vi "VIP_Post-Install Custom Action.vi"(10 "Variant":variant) -> (0 "error out":errorcluster)   [LabVIEW 2020]
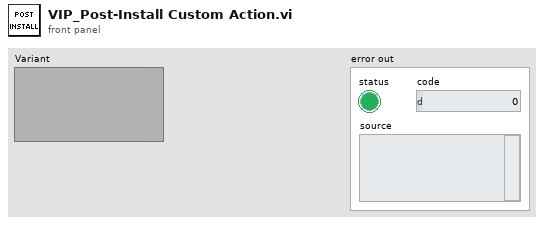
[diagram p1: front panel]
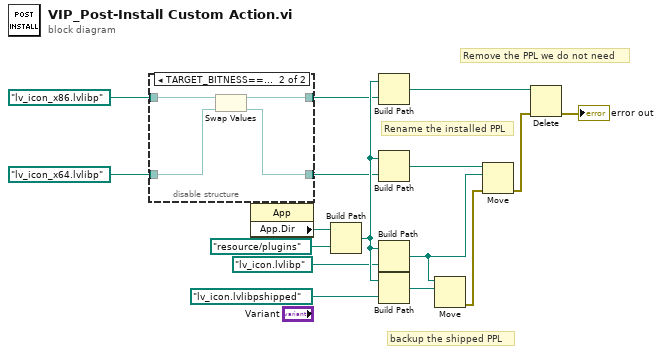
[diagram p0: block diagram]
diagram:
  # "Remove the PPL we do not need"
  # "Rename the installed PPL"
  # "backup the shipped PPL"
  n1 = disable-structure shown="TARGET_BITNESS==32" {
    disable-tunnel: path "lv_icon_x86.lvlibp" ("name or relative path") -> [w18 w22]
    disable-tunnel: [w18 w21] -> w3
    disable-tunnel: path "lv_icon_x64.lvlibp" ("name or relative path") -> [w17 w20]
    disable-tunnel: [w17 w19] -> w4
    frame condition #0 (active) {
    }
    frame condition #1 {
      n2 = Swap Values(12:w22, 14:w20) -> (1:w21:path, 3:w19:path)  [unwired: 1 in]
    }
  }
  n3 = property class="App"() -> ("App.Dir"=w1:path)  [unwired: 2 in, 2 out]
  n4 = Build Path(base path=w1, name or relative path=path "resource/plugins" ("symbolic path")) -> (appended path=w13:path)
  n5 = Build Path(base path=w13, name or relative path=w3) -> (appended path=w2:path)
  n6 = Build Path(base path=w13, name or relative path=w4) -> (appended path=w8:path)
  n7 = Build Path(base path=w13, name or relative path=path "lv_icon.lvlibp") -> (appended path=w9:path)
  n8 = Build Path(base path=w13, name or relative path=path "lv_icon.lvlibpshipped") -> (appended path=w7:path)
  n9 = Move(source path=w9, 10:w7) -> (error out=w16:errorcluster)  [unwired: 3 in, 2 out]
  n10 = Move(source path=w8, error in=w16, 10:w9) -> (error out=w15:errorcluster)  [unwired: 2 in, 2 out]
  n11 = Delete(path (use dialog)=w2, error in=w15) -> (error out=→"error out":errorcluster)  [unwired: 3 in, 2 out]
